vi "Initial Data.vi"(8 "error in (no error)":errorcluster, 11 "Masterv2 in":refnum<class "Masterv2.lvclass">) -> (0 "error out":errorcluster, 3 "Masterv2 out":refnum<class "Masterv2.lvclass">)   [LabVIEW 2014, in "Main Libraryv2.lvlib" / "Masterv2.lvclass"]
uses:
  Master/Masterv2.lvclass
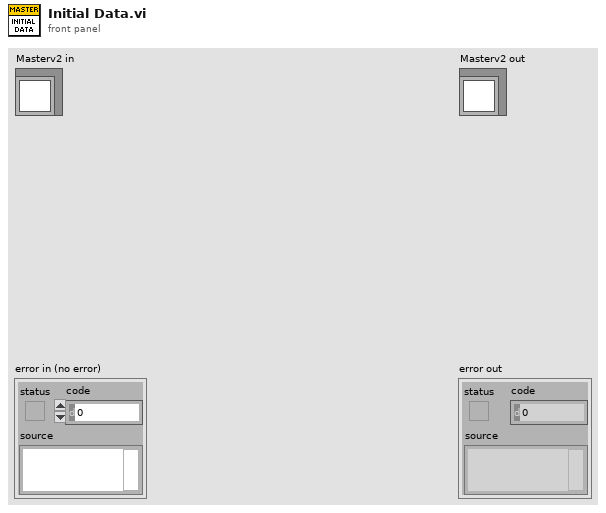
[diagram p1: front panel]
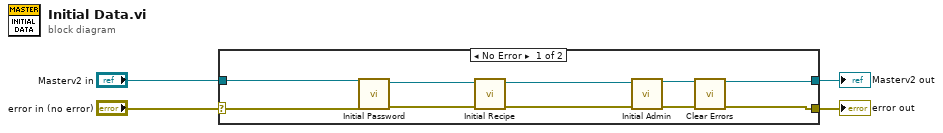
[diagram p0: block diagram]
diagram:
  n1 = case shown="No Error" "error in (no error)" {
    selector: "error in (no error)" -> [w13 w15]
    tunnel: [w9 w15] -> w3
    tunnel: [w5 w14] -> w1
    tunnel: "Masterv2 in" -> [w8 w14]
    frame No Error {
      n2 = call-dynamic "Initial Password.vi"("error in (no error)"=w13, "Masterv2 in"=w8) -> ("error out"=w12:errorcluster, "Masterv2 out"=w7:refnum<class "Masterv2.lvclass">)  [unwired: 8 in]
      n3 = call-dynamic "Initial Recipe.vi"("error in (no error)"=w12, "Masterv2 in"=w7) -> ("error out"=w11:errorcluster, "Masterv2 out"=w6:refnum<class "Masterv2.lvclass">)  [unwired: 8 in]
      n4 = call-dynamic "Initial Admin.vi"("error in (no error)"=w11, "Masterv2 in"=w6) -> ("error out"=w10:errorcluster, "Masterv2 out"=w5:refnum<class "Masterv2.lvclass">)  [unwired: 8 in]
      n5 = call <vilib>:"Clear Errors.vi"("error in (no error)"=w10) -> ("error out"=w9:errorcluster)  [unwired: 5 in, 1 out]
    }
    frame Error {
    }
  }
  "error out" <- w3
  "Masterv2 out" <- w1
